vi "Receive Reference (FPGA).vi"() -> ()   [LabVIEW 2019]
uses:
  SubVIs/Sync/Sync Control.ctl
  SubVIs/Sync/Sync Measurements.ctl
  <instrlib>/_niInstr/DSP/v1/Shared/Public/IQ Impairments.ctl
  <instrlib>/_niInstr/DSP/v1/Shared/Public/Filter Coefficients.ctl
  Host/SubVIs/Low-level/TypeDefs/Gain Setting.ctl
  <instrlib>/niMmWave/ni3620/Config/v1/FPGA/Public/Typedefs/TX1 RX1 Port.ctl
  <vilib>/Platform/TimedLoop/XDataNode/timing_clust.ctl
  <vilib>/Platform/TimedLoop/XDataNode/nitl_modes.ctl
  <vilib>/Platform/TimedLoop/XDataNode/wakeup.ctl
  <vilib>/rvi/Emulation/niFpgaSctlEmulationGetInTimedLoop.vi
  <vilib>/rvi/Emulation/niFpgaEmulationReportErrorSimple.vi
  <vilib>/rvi/Emulation/niFpgaGetClockAttributes.vi
  <vilib>/rvi/Emulation/niFpgaCriticalErrorInLSC.vi
  <vilib>/rvi/Emulation/niFpgaProcessEmulError.vi
  <vilib>/rvi/eio/common/nirviEmuTemplateMethod_errors.vi
  SubVIs/Misc/Globals.vi
  <instrlib>/_niInstr/Data Formatting/v1/FPGA/Private/Convert/U8 array to Boolean Array.vi
  <vilib>/rvi/Emulation/niFpgaEmulationIsFPGAContextNoSignature.vi
  <vilib>/rvi/errors/niFpgaSetErrorForExecOnDevCompSimple.vi
  <vilib>/rvi/eio/common/nirviEmuReportErrorAndStop.vi
  <vilib>/rvi/DataTransferAndStorage/Container/Common/niFpgaContainerGetUniqueNameForEmu.vi
  <vilib>/rvi/FIFO/Fifo_Resource/nirvififoEmulationSetSize.vi
  <vilib>/rvi/FIFO/Fifo_Resource/nirviFifoEmulationQueueMgr.vi
  <instcachedir>/0/nirviFifoEmulationQueueMgr_E5CAEC123FF24DC58D834DCA3CDAA9B5.lvgen/nirviFifoEmulationQueueMgr_E5CAEC123FF24DC58D834DCA3CDAA9B5_008.vi
  <vilib>/rvi/FIFO/Fifo_Resource/nirvififoEmulationDetermineInputValidOut.vi
  <vilib>/rvi/FIFO/Fifo_Resource/nirvififoEmulationCreateLock.vi
  <vilib>/rvi/FIFO/Fifo_Resource/nirvififoEmulationObtainLock.vi
  <vilib>/rvi/FIFO/Fifo_Resource/nirvififoEmulationReleaseLock.vi
  <vilib>/rvi/occurrence/nirviWaitOnOccurrenceBase.vi
  <vilib>/rvi/errors/nirviReportUnexpectedCaseInternalError.vi
  <vilib>/rvi/errors/nirviReportUnexpectedCaseInternalError (U32).vi
  <vilib>/rvi/interface/RandomDataEmulation/nirviRandomDataMultiElementFPGAFIFO.vi
  <instcachedir>/0/nirviRandomDataMultiElementFPGAFIFO_1ED88BA00AC641F388A9B1FAA20E354D.lvgen/nirviRandomDataMultiElementFPGAFIFO_1ED88BA00AC641F388A9B1FAA20E354D_003.vi
  <vilib>/rvi/interface/RandomDataEmulation/niFpgaRandomDataHandleErrors.vi
  <instrlib>/_niInstr/Basic Elements/v1/FPGA/Private/Count Down U32.vi
  <instrlib>/_niInstr/Basic Elements/v1/FPGA/Private/Count Up U8.vi
  <vilib>/rvi/DataTransferAndStorage/Container/Common/niFpgaContainerSetEmuInfo.vi
  <vilib>/Utility/error.llb/Clear Errors.vi
  <vilib>/Platform/TimedLoop/XDataNode/XDataNode.xnode
  <vilib>/eio/EIONode/EIONode.xnode
  <vilib>/eio/EIOMethodNode/EIOMethodNode.xnode
  <vilib>/rvi/DataTransferAndStorage/Container/XNode/niFpgaContainer.xnode
  <vilib>/rvi/FIFO/Fifo_Resource/nirvififoEmulationWrite.vi
  <vilib>/rvi/interface/RandomDataEmulation/nirviRandomDataFpgaMultiElementTemplate.vi
  <vilib>/rvi/LocalResourceManager/LocalResourceManager.xnode
  <vilib>/rvi/FIFO/Fifo_Resource/nirvififoEmulationRead.vi
  <vilib>/Platform/TimedLoop/XDataNode/XDNodeRunTimeDep.lvlib
  <instrlib>/_niInstr/Basic Elements/v1/FPGA/niInstr Basic Elements v1 FPGA.lvlib
  <instrlib>/_niInstr/Data Formatting/v1/FPGA/niInstr Data Formatting v1 FPGA.lvlib
  <instrlib>/niMmWave/ni3620/Config/v1/FPGA/niMmWave Config v1 FPGA.lvlib
  <instrlib>/_niInstr/DSP/v1/Shared/niInstr DSP v1 Shared.lvlib
panel:
  in  "sync.master reset listen":bool
  in  "sync.counter reset enable":bool
  in  "20 kHz tclk parameters":T1
  out "tclk value":u16
  in  "gain ranging.enable port config":bool
  out "port 5.debug info":T2
  out "port 5.rx fifo overflow":bool
  in  "port 5.rx fifo overflow clear":bool
  in  "aurora.read port 5":bool
  out "port 4.rx fifo overflow":bool
  in  "port 4.rx fifo overflow clear":bool
  out "port 4.debug info":T2
  in  "aurora.read port 4":bool
  in  "gain ranging.enable coarse gain ranging":bool
  in  "gain ranging.enable fine gain ranging":bool
  in  "gain ranging.coarse gain values":fxp<+/-,16,12>[](array[numeric])=[0.0, 0.0, 0.0, 0.0]
  in  "table info":T3
  in  "gain ranging.manual setting":T6
  in  "gain ranging.setting list step":T7
  in  "gain ranging.enable":bool
  in  "gain ranging.dwell time (cycles)":u32=4800
  in  "rxjesd.control":T8
  out "rxjesd.status":T9
  in  "filter.enable":bool
  in  "filter.coefficients":T10
  in  "cal.correction":T12={"sample delay"={"I delay"=0.0, "Q delay"=0.0}, "fractional delay"={"enable"=FALSE, "coef write"=FALSE, "coef data"=0.0}, "impairments"={"inline gain I"=0.9999923706054688, "inline gain Q"=0.9999923706054688, "cross gain I"=0.0, "cross gain Q"=0.0, "pre-gain offset I"=0.0, "pre-gain offset Q"=0.0, "post-gain offset I"=0.0, "post-gain offset Q"=0.0}, "iq inversion"={"invert I"=FALSE, "invert Q"=FALSE}}
  out "sync.measurements":T13
  in  "sync.parameters":T15
  in  "acq.length":u32=1024
  out "aurora.fifo 1 overflow":bool
  in  "aurora.reset trigger":bool=TRUE
  out "aurora.fifo 0 overflow":bool
  in  "aurora.write":bool
  in  "aurora.fifo overflow clear":bool
  out "clocks valid":bool[](array[boolean])
  in  "cal.acquisition":T16={"acq length"=1024, "trigger type"=enum."software", "software trigger"=FALSE, "reset trigger detect"=FALSE}
  in  "sync.use synced trigger":bool
  in  "sync.trigger":bool
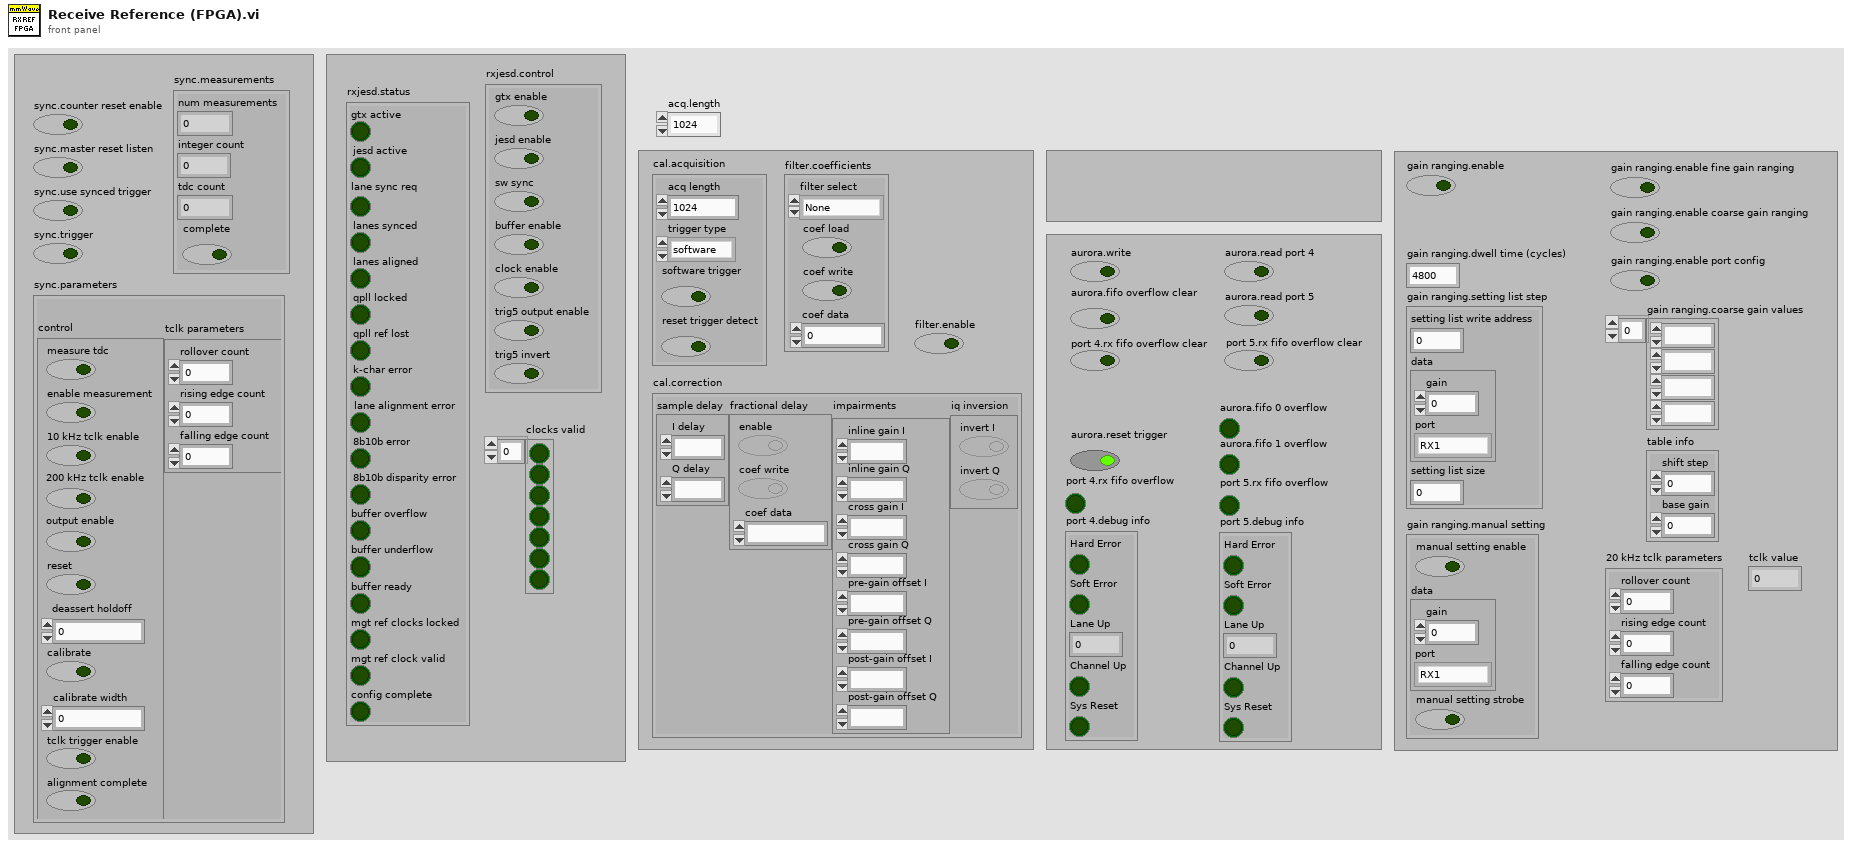
[diagram p1: front panel]
types:
  T1 = cluster{"rollover count":u16, "rising edge count":u16, "falling edge count":u16}
  T2 = cluster{"Hard Error":bool, "Soft Error":bool, "Lane Up":fxp<+,4,4>, "Channel Up":bool, "Sys Reset":bool}
  T3 = cluster{"shift step":i16, "base gain":fxp<+/-,16,12>}
  T4 = typedef "gain setting.ctl" = cluster{"gain":fxp<+/-,16,12>, "port":T5}
  T5 = typedef "TX1 RX1 Port.ctl" = enum8{"RX1", "TX1/RX2"}
  T6 = cluster{"manual setting enable":bool, "data":T4, "manual setting strobe":bool}
  T7 = cluster{"setting list write address":u32, "data":T4, "setting list size":u16}
  T8 = cluster{"gtx enable":bool, "jesd enable":bool, "sw sync":bool, "buffer enable":bool, "clock enable":bool, "trig5 output enable":bool, "trig5 invert":bool}
  T9 = cluster{"gtx active":bool, "jesd active":bool, "lane sync req":bool, "lanes synced":bool, "lanes aligned":bool, "qpll locked":bool, "qpll ref lost":bool, "k-char error":bool, "lane alignment error":bool, "8b10b error":bool, "8b10b disparity error":bool, "buffer overflow":bool, "buffer underflow":bool, "buffer ready":bool, "mgt ref clocks locked":bool, "mgt ref clock valid":bool, "config complete":bool}
  T10 = typedef "niInstr DSP v1 Shared.lvlib/Filter Coefficients.ctl" = cluster{"filter select":enum8{"None", "I Inline", "I Cross", "Q Cross", "Q Inline"}, "coef load":bool, "coef write":bool, "coef data":fxp<+/-,18,1>}
  T11 = typedef "niInstr DSP v1 Shared.lvlib/IQ Impairments.ctl" = cluster{"inline gain I":fxp<+/-,18,1>, "inline gain Q":fxp<+/-,18,1>, "cross gain I":fxp<+/-,18,1>, "cross gain Q":fxp<+/-,18,1>, "pre-gain offset I":fxp<+/-,18,1>, "pre-gain offset Q":fxp<+/-,18,1>, "post-gain offset I":fxp<+/-,18,1>, "post-gain offset Q":fxp<+/-,18,1>}
  T12 = cluster{"sample delay":cluster{"I delay":fxp<+,13,13>, "Q delay":fxp<+,13,13>}, "fractional delay":cluster{"enable":bool, "coef write":bool, "coef data":fxp<+/-,18,1>}, "impairments":T11, "iq inversion":cluster{"invert I":bool, "invert Q":bool}}
  T13 = typedef "Sync Measurements.ctl" = cluster{"num measurements":u16, "integer count":u16, "tdc count":u16, "complete":bool}
  T14 = typedef "Sync Control.ctl" = cluster{"measure tdc":bool, "enable measurement":bool, "10 kHz tclk enable":bool, "200 kHz tclk enable":bool, "output enable":bool, "reset":bool, "deassert holdoff":u8, "calibrate":bool, "calibrate width":u8, "tclk trigger enable":bool, "alignment complete":bool}
  T15 = cluster{"control":T14, "tclk parameters":cluster{"rollover count":u16, "rising edge count":u16, "falling edge count":u16}}
  T16 = cluster{"acq length":u16, "trigger type":enum16{"software", "external", "rising zero", "falling zero"}, "software trigger":bool, "reset trigger detect":bool}
  T17 = cluster{"m_axis_tvalid":refnum<k21>, "m_axis_tdata_0":refnum<k21>, "m_axis_tdata_1":refnum<k21>, "m_axis_tdata_2":refnum<k21>, "m_axis_tdata_3":refnum<k21>}
  T18 = cluster{"s_axis_tvalid":refnum<k21>, "s_axis_tdata_0":refnum<k21>, "s_axis_tdata_1":refnum<k21>, "s_axis_tdata_2":refnum<k21>, "s_axis_tdata_3":refnum<k21>, "s_axis_tready":refnum<k21>}
  T19 = typedef "Sync Resources.ctl" = cluster{"tdc assert":refnum<k21>, "tdc deassert":refnum<k21>, "tdc count":refnum<k21>, "control":refnum<k21>, "integer count":refnum<k21>}
  T20 = typedef "XDNodeRunTimeDep.lvlib/timing_clust.ctl" = cluster{"Expected End [f-1]":u64, "Actual End [f-1]":u64, "Finished Late? [f-1]":bool, "Expected End [i-1]":u64, "Actual End [i-1]":u64, "Finished Late? [i-1]":bool, "Expected Start [i]":u64, "Actual Start [i]":u64, "Expected Start [f]":u64, "Actual Start [f]":u64, "Source Name":string, "Structure Name":string, "Period":i64, "Deadline":i64, "Offset":i64, "Start":i64, "Priority":i32, "Timeout":i32, "Mode":T21, "Wakeup Reason":T22, "Error":errorcluster, "Source Type":string, "Secondary Source Type":string, "Global End Time":u64, "Global Start Time":u64, "Frame Duration":u64, "Iteration Duration":u64, "Assigned CPU":i32, "I/O Scan Engine Mode":u32}
  T21 = typedef "XDNodeRunTimeDep.lvlib/nitl_modes.ctl" = enum32{"No Change", "Process missed periods, maintain original phase", "Discard missed periods, maintain original phase", "Process missed periods, ignore original phase", "Discard missed periods, ignore original phase"}
  T22 = typedef "XDNodeRunTimeDep.lvlib/wakeup.ctl" = enum32{"Normal", "Aborted", "Asynchronous wakeup", "Timing source error", "Timed loop error", "Timeout"}
  T23 = cluster{"disable TClk measure":bool, "output enable":bool, "output value":bool}
  T24 = typedef "niInstr DSP v1 Shared.lvlib/IQ Data.ctl" = cluster{"I":fxp<+/-,18,1>, "Q":fxp<+/-,18,1>, "overflow":bool}
  T25 = typedef "AXI4-Stream Reader FXP64x4 Resources.ctl" = cluster{"AXI4-Stream Reader Resources":cluster{"Use TREADY":bool, "Use TLAST":bool, "TLAST":refnum<k21>, "TREADY":refnum<k21>, "TVALID":refnum<k21>, "Use TKEEP":bool, "Use TSTRB":bool, "Use TUSER":bool}, "TDATA Resources":cluster{"TDATA_0":refnum<k21>, "TDATA_1":refnum<k21>, "TDATA_2":refnum<k21>, "TDATA_3":refnum<k21>}, "TKEEP":refnum<k21>, "TSTRB":refnum<k21>}
  T26 = typedef "AXI4-Stream Writer FXP64x4 Resources.ctl" = cluster{"Writer Resources":cluster{"Use TREADY":bool, "Use TLAST":bool, "TLAST":refnum<k21>, "TREADY":refnum<k21>, "TVALID":refnum<k21>, "Use TSTRB":bool, "Use TKEEP":bool, "Use TUSER":bool}, "TDATA Resources":cluster{"TDATA_0":refnum<k21>, "TDATA_1":refnum<k21>, "TDATA_2":refnum<k21>, "TDATA_3":refnum<k21>}, "TKEEP":refnum<k21>, "TSTRB":refnum<k21>}
  T27 = cluster{"Hard Error":refnum<k21>, "Soft Error":refnum<k21>, "Lane Up":refnum<k21>, "Channel Up":refnum<k21>, "Sys Reset":refnum<k21>}
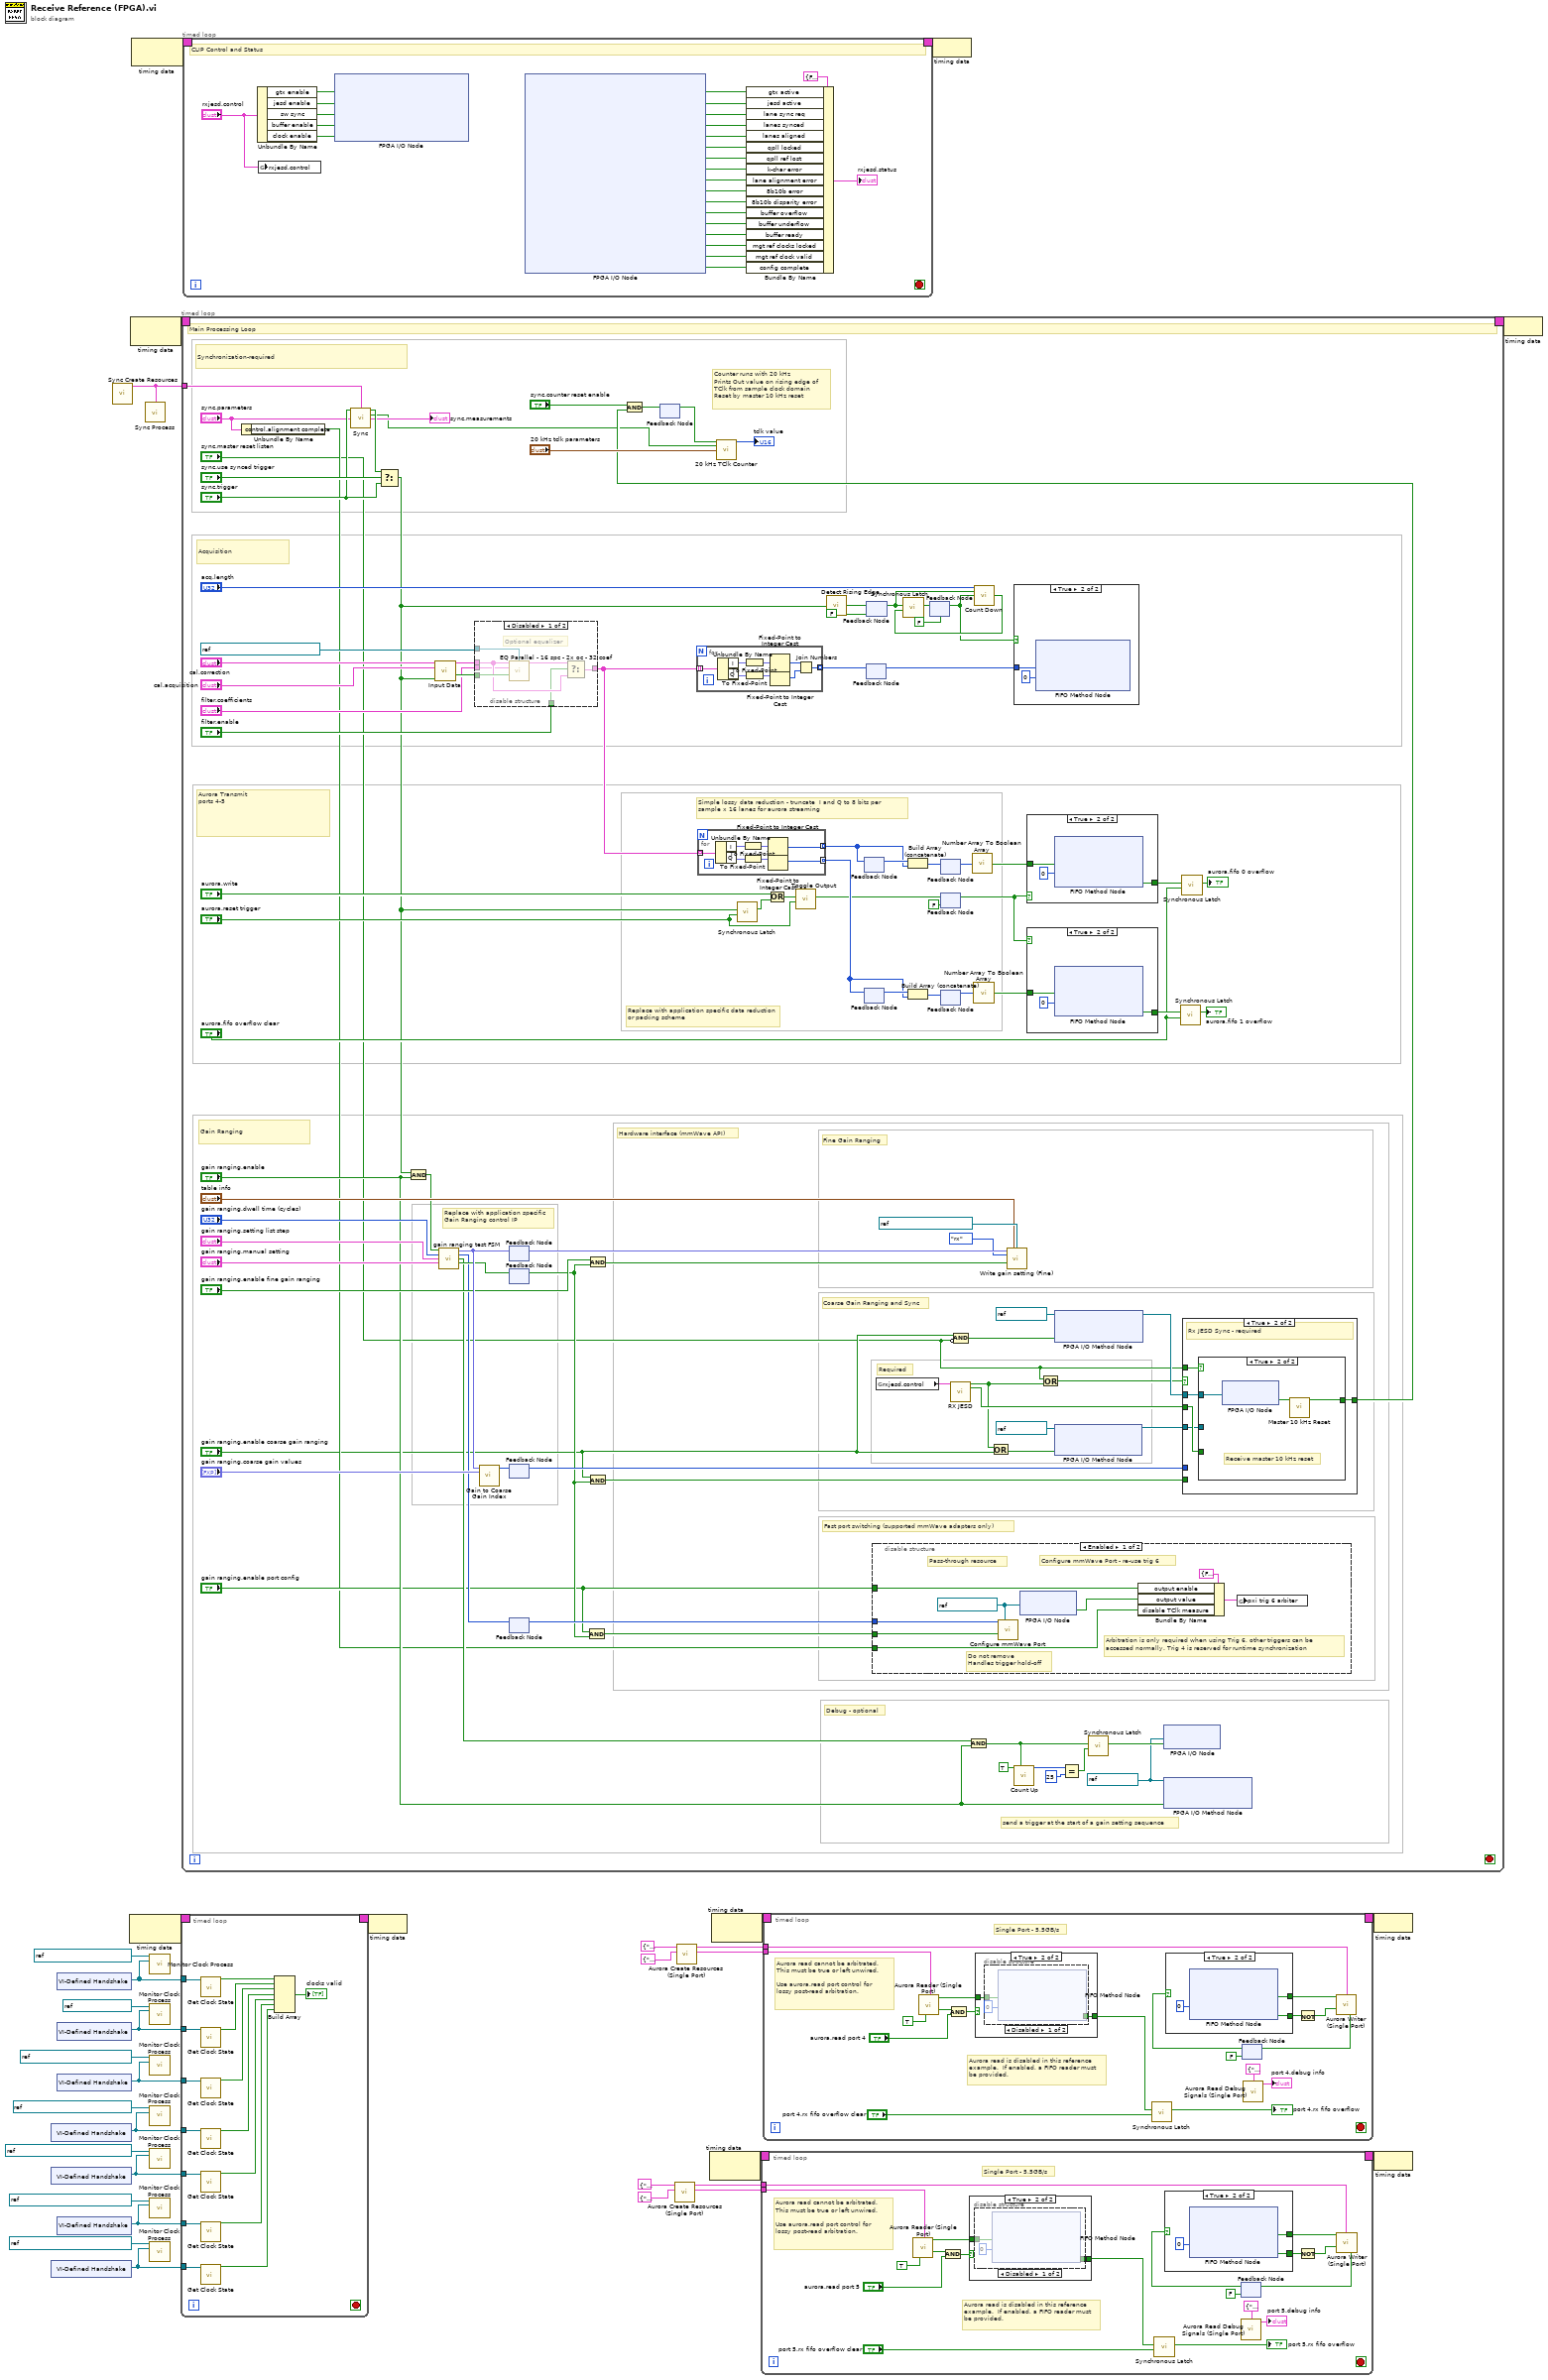
[diagram p0: block diagram]
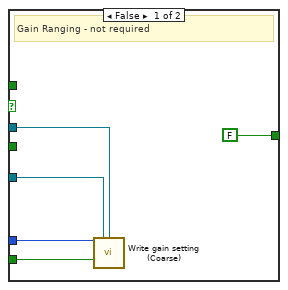
[diagram p2: hidden frame]
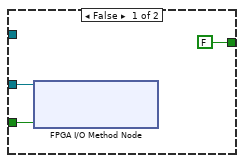
[diagram p3: hidden frame]
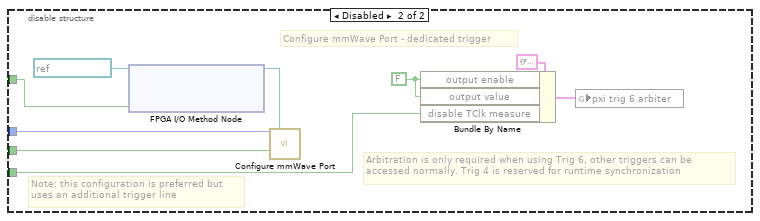
[diagram p4: hidden frame]
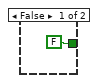
[diagram p7: hidden frame]
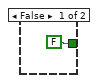
[diagram p8: hidden frame]
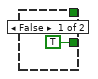
[diagram p9: hidden frame]
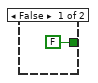
[diagram p10: hidden frame]
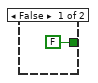
[diagram p12: hidden frame]
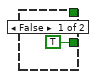
[diagram p14: hidden frame]
diagram:
  n1 = xnode "VI-Defined Handshake"() -> ("Handshake Out"=w10:refnum<k21>)
  n2 = xnode "VI-Defined Handshake"() -> ("Handshake Out"=w11:refnum<k21>)
  n3 = xnode "VI-Defined Handshake"() -> ("Handshake Out"=w18:refnum<k21>)
  n4 = xnode "VI-Defined Handshake"() -> ("Handshake Out"=w25:refnum<k21>)
  n5 = xnode "VI-Defined Handshake"() -> ("Handshake Out"=w24:refnum<k21>)
  n6 = xnode "VI-Defined Handshake"() -> ("Handshake Out"=w20:refnum<k21>)
  n7 = xnode "VI-Defined Handshake"() -> ("Handshake Out"=w21:refnum<k21>)
  n8 = call "Sync Create Resources.vi"() -> ("sync.resources"=w29:T19)  [unwired: 15 in]
  n9 = node-c288() -> (w28:T20)  [unwired: 1 in]
  n10 = node-c288() -> (w31:T20)  [unwired: 1 in]
  n11 = node-c288() -> (w33:T20)  [unwired: 1 in]
  n12 = call "Sync Process.vi"("sync.resources"=w29) -> ()  [unwired: 15 in]
  n13 = call "Monitor Clock Process.vi"("clock name"=refnum<k21> "40 MHz Onboard Clock", "handshake"=w25) -> ()  [unwired: 14 in]
  n14 = call "Monitor Clock Process.vi"("clock name"=refnum<k21> "100 MHz Clock", "handshake"=w24) -> ()  [unwired: 14 in]
  n15 = call "Monitor Clock Process.vi"("clock name"=refnum<k21> "7902R IO Socket\\SampleClk", "handshake"=w20) -> ()  [unwired: 14 in]
  n16 = call "Monitor Clock Process.vi"("clock name"=refnum<k21> "7902R IO Socket\\SampleClkx2", "handshake"=w10) -> ()  [unwired: 14 in]
  n17 = call "Monitor Clock Process.vi"("clock name"=refnum<k21> "7902R IO Socket\\SampleClkDiv2", "handshake"=w11) -> ()  [unwired: 14 in]
  n18 = call "Monitor Clock Process.vi"("clock name"=refnum<k21> "7902R IO Socket\\Port4_UserClk", "handshake"=w21) -> ()  [unwired: 14 in]
  n19 = call "Monitor Clock Process.vi"("clock name"=refnum<k21> "7902R IO Socket\\Port5_UserClk", "handshake"=w18) -> ()  [unwired: 14 in]
  n20 = timed-loop {
    timing: w28 -> [_]
    timing-out: [_] -> w27
    tunnel: w25 -> [w48]
    tunnel: w24 -> [w47]
    tunnel: w20 -> [w42]
    tunnel: w21 -> [w43]
    tunnel: w18 -> [w40]
    tunnel: w10 -> [w38]
    tunnel: w11 -> [w39]
    stop <- _ stop-if-true
    n21 = call "Get Clock State.vi"("handshake in"=w48) -> ("clock valid"=w46:bool)  [unwired: 14 in]
    n22 = call "Get Clock State.vi"("handshake in"=w47) -> ("clock valid"=w45:bool)  [unwired: 14 in]
    n23 = call "Get Clock State.vi"("handshake in"=w42) -> ("clock valid"=w41:bool)  [unwired: 14 in]
    n24 = call "Get Clock State.vi"("handshake in"=w38) -> ("clock valid"=w35:bool)  [unwired: 14 in]
    n25 = call "Get Clock State.vi"("handshake in"=w39) -> ("clock valid"=w34:bool)  [unwired: 14 in]
    n26 = call "Get Clock State.vi"("handshake in"=w43) -> ("clock valid"=w36:bool)  [unwired: 14 in]
    n27 = call "Get Clock State.vi"("handshake in"=w40) -> ("clock valid"=w37:bool)  [unwired: 14 in]
    n28 = Build Array(w46, w45, w41, w35, w34, w36, w37) -> (→"clocks valid":bool[])
  }
  n29 = timed-loop {
    timing: w31 -> [_]
    timing-out: [_] -> w30
    tunnel: w29 -> [w123]
    stop <- _ stop-if-true
    w80 = refnum<k21> "PXI_Trig3" ("FPGA I/O In")
    # "Counter runs with 20 kHz\nPrints Out value on rising edge of \nTClk from sample clock domain\nReset by master 10 kHz reset"
    # "Replace with application specific Gain Ranging control IP"
    # "Simple lossy data reduction - truncate  I and Q to 8 bits per sample x 16 lanes for aurora streaming"
    # "Replace with application specific data reduction or packing scheme"
    # "Debug - optional"
    # "Fast port switching (supported mmWave adapters only)"
    # "Coarse Gain Ranging and Sync"
    # "Fine Gain Ranging"
    # "Hardware interface (mmWave API)"
    # "Gain Ranging"
    # "Aurora Transmit\nports 4-5"
    # "Acquisition"
    # "Synchronization-required"
    # "Required"
    # "send a trigger at the start of a gain setting sequence"
    # "Main Processing Loop"
    n30 = Unbundle By Name("sync.parameters") -> ("control.alignment complete"=w63:bool)
    n31 = call "Sync.vi"("trigger"="sync.trigger", "sync.resources"=w123, "sync.parameters"="sync.parameters") -> ("synced trigger"=w124:bool, "tclk"=w54:bool, "sync measurements"=→"sync.measurements":T13)  [unwired: 10 in]
    n32 = Select(t=w124, s="sync.use synced trigger", f="sync.trigger") -> (s? t:f=w101:bool)
    n33 = And(x=w101, y="gain ranging.enable") -> (x .and. y?=w78:bool)
    n34 = call "Input Data.vi"("cal parameters"="cal.correction", "acq parameters"="cal.acquisition", "external trigger"=w101) -> ("adc data"=w108:T24[], "output valid"=w110:bool)  [unwired: 11 in]
    n35 = call "gain ranging test FSM.vi"("gain ranging.start sequence"=w78, "gain ranging.dwell time (cycles)"="gain ranging.dwell time (cycles)", "gain ranging.gain setting list"="gain ranging.setting list step", "gain ranging.manual request"="gain ranging.manual setting") -> ("gain ranging.gain setting"=w95:fxp<+/-,16,12>, "gain ranging.TX1/RX1 Port Value"=w88:T5, "gain ranging.start of sequence"=w86:bool, "gain ranging.gain setting valid"=w90:bool)  [unwired: 8 in]
    n36 = disable-structure shown="Disabled" {
      disable-tunnel: w110 -> [w187 _]
      disable-tunnel: [w185 w188] -> w109
      disable-tunnel: w108 -> [w184 w188]
      disable-tunnel: "filter.coefficients" -> [w183 _]
      disable-tunnel: "filter.enable" -> [w182 _]
      disable-tunnel: refnum<k21> "7902R IO Socket\\SampleClkx2" ("clock x2") -> [w181 _]
      frame Disabled {
        # "Optional equalizer"
        n37 = call "EQ Parallel - 16 spc - 2x oc - 32 coef.vi"("data in"=w184, "clock x2"=w181, "filter coefficients"=w183, "input valid"=w187) -> ("data out"=w186:T24[])  [unwired: 9 in, 2 out]
        n38 = Select(t=w186, s=w182, f=w184) -> (s? t:f=w185:T24[])
      }
      frame Enabled {
      }
    }
    n39 = call "Gain to Coarse Gain Index.vi"("gain setting"=w95, "coarse gain values"="gain ranging.coarse gain values") -> ("coarse gain index"=w93:u32)  [unwired: 13 in]
    n40 = feedback #1() -> (w94:fxp<+/-,16,12>)  [unwired: 1 in]
    n41 = feedback-in #1(w95) -> ()
    n42 = feedback #2() -> (w68:bool)  [unwired: 1 in]
    n43 = feedback-in #2(w90) -> ()
    n44 = feedback #3() -> (w71:u32)  [unwired: 1 in]
    n45 = feedback-in #3(w93) -> ()
    n46 = feedback #4() -> (w76:T5)  [unwired: 1 in]
    n47 = feedback-in #4(w88) -> ()
    n48 = And(x="gain ranging.enable port config", y=w68) -> (x .and. y?=w67:bool)
    n49 = And(x="gain ranging.enable fine gain ranging", y=w68) -> (x .and. y?=w89:bool)
    n50 = And(x="gain ranging.enable coarse gain ranging", y=w68) -> (x .and. y?=w70:bool)
    n51 = feedback #5() -> (w55:bool)  [unwired: 1 in]
    n52 = for {
      tunnel: [w196] -> w112 mode=indexing
      tunnel: w109 -> [w195] mode=indexing
      n53 = Unbundle By Name(w195) -> ("I"=w194:fxp<+/-,18,1>, "Q"=w193:fxp<+/-,18,1>)
      n54 = To Fixed-Point(number=w194) -> (fixed-point=w198:fxp<+/-,16,1>)  [unwired: 1 in]
      n55 = To Fixed-Point(number=w193) -> (fixed-point=w197:fxp<+/-,16,1>)  [unwired: 1 in]
      n56 = Fixed-Point to Integer Cast(1:w198) -> (0:w192:i16)
      n57 = Fixed-Point to Integer Cast(1:w197) -> (0:w191:i16)
      n58 = Join Numbers(hi=w192, lo=w191) -> ((hi.lo)=w196:u32)
    }
    n59 = for {
      tunnel: w109 -> [w211] mode=indexing
      tunnel: [w208] -> w117 mode=indexing
      tunnel: [w207] -> w120 mode=indexing
      n60 = Unbundle By Name(w211) -> ("I"=w210:fxp<+/-,18,1>, "Q"=w209:fxp<+/-,18,1>)
      n61 = To Fixed-Point(number=w210) -> (fixed-point=w213:fxp<+/-,8,1>)  [unwired: 1 in]
      n62 = To Fixed-Point(number=w209) -> (fixed-point=w212:fxp<+/-,8,1>)  [unwired: 1 in]
      n63 = Fixed-Point to Integer Cast(1:w213) -> (0:w208:i8)
      n64 = Fixed-Point to Integer Cast(1:w212) -> (0:w207:i8)
    }
    n65 = call "20 kHz TClk Counter.vi"("master 10 kHz reset"=w55, "tclk"=w54, "20 kHz tclk parameters"="20 kHz tclk parameters") -> ("tclk offset value"=→"tclk value":u16)  [unwired: 12 in]
    n66 = call <instrlib>:"Synchronous Latch.vi"("clear"="aurora.reset trigger", "set"=w101) -> ("out"=w140:bool)  [unwired: 9 in]
    n67 = Or(x="aurora.write", y=w140) -> (x .or. y?=w115:bool)
    n68 = call <instrlib>:"Toggle Output.vi"("clear"="aurora.reset trigger", "toggle"=w115) -> ("output"=w114:bool)  [unwired: 9 in]
    n69 = call <instrlib>:"Detect Rising Edge.vi"("signal"=w101) -> ("edge detected"=w129:bool)  [unwired: 14 in]
    n70 = feedback #6() -> (w118:i8[])  [unwired: 1 in]
    n71 = feedback-in #6(w117) -> ()
    n72 = feedback #7() -> (w121:i8[])  [unwired: 1 in]
    n73 = feedback-in #7(w120) -> ()
    n74 = feedback #8() -> (w128:u32[])  [unwired: 1 in]
    n75 = feedback-in #8(w112) -> ()
    n76 = feedback #9(FALSE ("edge detected")) -> (w130:bool)
    n77 = feedback-in #9(w129) -> ()
    n78 = disable-structure shown="Enabled" {
      disable-tunnel: w67 -> [w169 w178]
      disable-tunnel: w76 -> [w168 w177]
      disable-tunnel: "gain ranging.enable port config" -> [w166 w174]
      disable-tunnel: w63 -> [w164 w172]
      frame Enabled {
        w165 = refnum<k21> "PXIe_DStarC" ("FPGA I/O In")
        # "Do not remove\nHandles trigger hold-off"
        # "Configure mmWave Port - re-use trig 6"
        # "Pass-through resource"
        # "Arbitration is only required when using Trig 6, other triggers can be accessed normally. Trig 4 is reserved for runtime synchronization"
        n79 = call <instrlib>:"Configure mmWave Port.vi"("port"=w168, "pxi trigger"=w165, "input valid"=w169) -> ()  [unwired: 12 in, 1 out]
        n80 = xnode "FPGA I/O Node"("FPGA I/O In"=w165) -> ("I/O Item"=w167:bool)  [unwired: 1 out]
        n81 = Bundle By Name(cluster=T23 {"disable TClk measure"=FALSE, "output enable"=FALSE, "output value"=FALSE} ("pxi trig 6 arbiter"), "output enable"=w166, "output value"=w167, "disable TClk measure"=w164) -> (w170:T23)
        n82 = global write "Globals.vi" "pxi trig 6 arbiter"(w170) -> ()
      }
      frame Disabled {
        w176 = FALSE ("disable TClk measure")
        # "Note: this configuration is preferred but \nuses an additional trigger line"
        # "Configure mmWave Port - dedicated trigger"
        # "Arbitration is only required when using Trig 6, other triggers can be accessed normally. Trig 4 is reserved for runtime synchronization"
        n83 = xnode "FPGA I/O Method Node"("FPGA I/O In"=refnum<k21> "PXI_Trig0" ("pxi trigger 1"), "Enable"=w174) -> ("FPGA I/O Out"=w175:refnum<k21>)
        n84 = call <instrlib>:"Configure mmWave Port.vi"("port"=w177, "pxi trigger"=w175, "input valid"=w178) -> ()  [unwired: 12 in, 1 out]
        n85 = Bundle By Name(cluster=T23 {"disable TClk measure"=FALSE, "output enable"=FALSE, "output value"=FALSE} ("pxi trig 6 arbiter"), "output enable"=w176, "output value"=w176, "disable TClk measure"=w172) -> (w179:T23)
        n86 = global write "Globals.vi" "pxi trig 6 arbiter"(w179) -> ()
      }
    }
    n87 = global read "Globals.vi" "rxjesd.control"() -> (w97:T8)
    n88 = Build Array (concatenate)(w118, w117) -> (w116:i8[])
    n89 = Build Array (concatenate)(w121, w120) -> (w119:i8[])
    n90 = feedback #10(FALSE ("out")) -> (w125:bool)
    n91 = feedback #11() -> (w142:i8[])  [unwired: 1 in]
    n92 = feedback-in #11(w116) -> ()
    n93 = feedback #12(FALSE) -> (w138:bool)
    n94 = feedback-in #12(w114) -> ()
    n95 = feedback #13() -> (w137:i8[])  [unwired: 1 in]
    n96 = feedback-in #13(w119) -> ()
    n97 = call "RX JESD.vi"("rxjesd.control"=w97) -> ("trigger output enable"=w53:bool, "trigger value"=w73:bool)  [unwired: 13 in]
    n98 = Compound Arithmetic op=AND("gain ranging.enable coarse gain ranging", invert "sync.master reset listen") -> (w61:bool)
    n99 = And(x=w86, y="gain ranging.enable") -> (x .and. y?=w79:bool)
    n100 = call-poly <instrlib>:"Number Array To Boolean Array.vi"("data in"=w142) -> ("data out"=w145:bool[])  [unwired: 14 in]
    n101 = call-poly <instrlib>:"Number Array To Boolean Array.vi"("data in"=w137) -> ("data out"=w136:bool[])  [unwired: 14 in]
    n102 = call-poly <instrlib>:"Count Down.vi"("count in"="acq.length", "load"=w130, "decrement"=w125) -> ("terminal count"=w126:bool)  [unwired: 11 in, 1 out]
    n103 = call <instrlib>:"Synchronous Latch.vi"("clear"=w126, "set"=w130) -> ("out"=w127:bool)  [unwired: 9 in]
    n104 = feedback-in #10(w127) -> ()
    n105 = Or(x=w53, y="gain ranging.enable coarse gain ranging") -> (x .or. y?=w69:bool)
    n106 = call <instrlib>:"Write gain setting (Fine).vi"("gain"=w94, "table info"="table info", "P2P Writer FIFO"=refnum<k21> "P2P FIFO to PXIe-3620" ("FIFO In"), "direction"=enum8{"rx", "tx"}."rx", "input valid"=w89) -> ()  [unwired: 10 in, 1 out]
    n107 = case shown="True" w125 {
      tunnel: w128 -> [_ w190]
      frame False {
      }
      frame True {
        n108 = xnode ("FIFO Method Node")("Element"=w190, "Timeout"=0) -> ()  [unwired: 1 in, 2 out]
      }
    }
    n109 = call-poly <instrlib>:"Count Up.vi"("increment"=TRUE, "reset"=w79) -> ("count out"=w84:u8)  [unwired: 13 in]
    n110 = case shown="True" w138 {
      tunnel: [FALSE ("Timed Out?") w206] -> w143
      tunnel: w145 -> [_ w205]
      frame False {
      }
      frame True {
        n111 = xnode ("FIFO Method Node")("Element"=w205, "Timeout"=0) -> ("Timed Out?"=w206:bool)  [unwired: 1 in, 1 out]
      }
    }
    n112 = case shown="True" w138 {
      tunnel: [FALSE ("Timed Out?") w202] -> w134
      tunnel: w136 -> [_ w201]
      frame False {
      }
      frame True {
        n113 = xnode ("FIFO Method Node")("Element"=w201, "Timeout"=0) -> ("Timed Out?"=w202:bool)  [unwired: 1 in, 1 out]
      }
    }
    n114 = Or(x="sync.master reset listen", y=w53) -> (x .or. y?=w52:bool)
    n115 = xnode "FPGA I/O Method Node"("FPGA I/O In"=refnum<k21> "PXI_Trig5" ("pxi trigger 1"), "Enable"=w69) -> ("FPGA I/O Out"=w72:refnum<k21>)
    n116 = xnode "FPGA I/O Method Node"("FPGA I/O In"=refnum<k21> "PXI_Trig7" ("pxi trigger 1"), "Enable"=w61) -> ("FPGA I/O Out"=w74:refnum<k21>)
    n117 = Equal?(x=w84, y=u8 25) -> (x = y?=w82:bool)
    n118 = call <instrlib>:"Synchronous Latch.vi"("clear"=w82, "set"=w79) -> ("out"=w81:bool)  [unwired: 9 in]
    n119 = xnode "FPGA I/O Node"("I/O Item"=w81, "FPGA I/O In"=w80) -> ()  [unwired: 1 out]
    n120 = xnode "FPGA I/O Method Node"("FPGA I/O In"=w80, "Enable"="gain ranging.enable") -> ()  [unwired: 1 out]
    n121 = call <instrlib>:"Synchronous Latch.vi"("clear"="aurora.fifo overflow clear", "set"=w134) -> ("out"=→"aurora.fifo 1 overflow":bool)  [unwired: 9 in]
    n122 = call <instrlib>:"Synchronous Latch.vi"("clear"="aurora.fifo overflow clear", "set"=w143) -> ("out"=→"aurora.fifo 0 overflow":bool)  [unwired: 9 in]
    n123 = case shown="True" w52 {
      tunnel: w74 -> [w152 w153]
      tunnel: w73 -> [_ w157]
      tunnel: w72 -> [w151 w156]
      tunnel: w71 -> [w150 _]
      tunnel: w70 -> [w149 _]
      tunnel: [FALSE ("Master10k_Reset") w155] -> w58
      tunnel: "sync.master reset listen" -> [_ w154]
      frame False {
        # "Gain Ranging - not required"
        n124 = call <instrlib>:"Write gain setting (Coarse).vi"("fast jump table index"=w150, "pxi trigger 1"=w151, "pxi trigger 2"=w152, "input valid"=w149) -> ()  [unwired: 11 in, 1 out]
      }
      frame True {
        # "Rx JESD Sync - required"
        n125 = case shown="True" w154 {
          tunnel: w157 -> [w160 _]
          tunnel: w156 -> [w159 _]
          tunnel: [FALSE ("Master10k_Reset") w161] -> w155
          tunnel: w153 -> [_ w162]
          frame False {
            n126 = xnode "FPGA I/O Method Node"("FPGA I/O In"=w159, "Data"=w160) -> ()  [unwired: 1 out]
          }
          frame True {
            # "Receive master 10 kHz reset"
            n127 = xnode "FPGA I/O Node"("FPGA I/O In"=w162) -> ("I/O Item"=w163:bool)  [unwired: 1 out]
            n128 = call "Master 10 kHz Reset.vi"("I/O Item"=w163) -> ("master 10 kHz reset"=w161:bool)  [unwired: 10 in]
          }
        }
      }
    }
    n129 = And(x="sync.counter reset enable", y=w58) -> (x .and. y?=w57:bool)
    n130 = feedback-in #5(w57) -> ()
  }
  n131 = timed-loop {
    timing: w33 -> [_]
    timing-out: [_] -> w32
    stop <- _ stop-if-true
    # "CLIP Control and Status"
    n132 = Unbundle By Name("rxjesd.control") -> ("gtx enable"=w218:bool, "jesd enable"=w222:bool, "sw sync"=w221:bool, "buffer enable"=w220:bool, "clock enable"=w217:bool)
    n133 = global write "Globals.vi" "rxjesd.control"("rxjesd.control") -> ()
    n134 = xnode "FPGA I/O Node"("7902R IO Socket\\aGtxEnable"=w218, "7902R IO Socket\\aJesdEnable"=w222, "7902R IO Socket\\aSyncFromSw"=w221, "7902R IO Socket\\aBufferEnable"=w220, "7902R IO Socket\\aClkEnable"=w217) -> ()  [unwired: 5 in, 5 out]
    n135 = xnode "FPGA I/O Node"() -> ("7902R IO Socket\\aGtxActive"=w216:bool, "7902R IO Socket\\aJesdActive"=w239:bool, "7902R IO Socket\\aLaneSyncReq"=w238:bool, "7902R IO Socket\\aLanesSynced"=w237:bool, "7902R IO Socket\\aLanesAligned"=w236:bool, "7902R IO Socket\\aQpllLocked"=w235:bool, "7902R IO Socket\\aQpllRefLost"=w234:bool, "7902R IO Socket\\aKCharError"=w233:bool, "7902R IO Socket\\aLaneAlignError"=w232:bool, "7902R IO Socket\\a8b10bNotInTable"=w231:bool, "7902R IO Socket\\a8b10bDispError"=w230:bool, "7902R IO Socket\\aBufferOverflow"=w229:bool, "7902R IO Socket\\aBufferUnderflow"=w228:bool, "7902R IO Socket\\aBufferReady"=w227:bool, "7902R IO Socket\\MgtRefClks_Locked"=w226:bool, "7902R IO Socket\\MgtRefClks_Valid"=w225:bool, "7902R IO Socket\\sFrontEndConfig_Complete"=w224:bool)  [unwired: 17 in, 17 out]
    n136 = Bundle By Name(cluster=T9 {"gtx active"=FALSE, "jesd active"=FALSE, "lane sync req"=FALSE, "lanes synced"=FALSE, "lanes aligned"=FALSE, "qpll locked"=FALSE, "qpll ref lost"=FALSE, "k-char error"=FALSE, "lane alignment error"=FALSE, "8b10b error"=FALSE, "8b10b disparity error"=FALSE, "buffer overflow"=FALSE, "buffer underflow"=FALSE, "buffer ready"=FALSE, "mgt ref clocks locked"=FALSE, "mgt ref clock valid"=FALSE, "config complete"=FALSE} ("rxjesd.status 2"), "gtx active"=w216, "jesd active"=w239, "lane sync req"=w238, "lanes synced"=w237, "lanes aligned"=w236, "qpll locked"=w235, "qpll ref lost"=w234, "k-char error"=w233, "lane alignment error"=w232, "8b10b error"=w231, "8b10b disparity error"=w230, "buffer overflow"=w229, "buffer underflow"=w228, "buffer ready"=w227, "mgt ref clocks locked"=w226, "mgt ref clock valid"=w225, "config complete"=w224) -> (→"rxjesd.status":T9)
  }
  n137 = node-c288(w27) -> ()
  n138 = call "Aurora Create Resources (Single Port).vi"("RX CLIP Resources"=T17 {"m_axis_tvalid"="7902R IO Socket\\uPort5_m_axi_rx_tvalid", "m_axis_tdata_0"="7902R IO Socket\\uPort5_m_axi_rx_tdata_0", "m_axis_tdata_1"="7902R IO Socket\\uPort5_m_axi_rx_tdata_1", "m_axis_tdata_2"="7902R IO Socket\\uPort5_m_axi_rx_tdata_2", "m_axis_tdata_3"="7902R IO Socket\\uPort5_m_axi_rx_tdata_3"}, "TX CLIP Resources"=T18 {"s_axis_tvalid"="7902R IO Socket\\uPort5_s_axi_tx_tvalid", "s_axis_tdata_0"="7902R IO Socket\\uPort5_s_axi_tx_tdata_0", "s_axis_tdata_1"="7902R IO Socket\\uPort5_s_axi_tx_tdata_1", "s_axis_tdata_2"="7902R IO Socket\\uPort5_s_axi_tx_tdata_2", "s_axis_tdata_3"="7902R IO Socket\\uPort5_s_axi_tx_tdata_3", "s_axis_tready"="7902R IO Socket\\uPort5_s_axi_tx_tready"}) -> ("AXI4-Stream Reader FXP64x4"=w3:T25, "AXI4-Stream Writer FXP64x4"=w4:T26)  [unwired: 8 in]
  n139 = call "Aurora Create Resources (Single Port).vi"("RX CLIP Resources"=T17 {"m_axis_tvalid"="7902R IO Socket\\uPort4_m_axi_rx_tvalid", "m_axis_tdata_0"="7902R IO Socket\\uPort4_m_axi_rx_tdata_0", "m_axis_tdata_1"="7902R IO Socket\\uPort4_m_axi_rx_tdata_1", "m_axis_tdata_2"="7902R IO Socket\\uPort4_m_axi_rx_tdata_2", "m_axis_tdata_3"="7902R IO Socket\\uPort4_m_axi_rx_tdata_3"}, "TX CLIP Resources"=T18 {"s_axis_tvalid"="7902R IO Socket\\uPort4_s_axi_tx_tvalid", "s_axis_tdata_0"="7902R IO Socket\\uPort4_s_axi_tx_tdata_0", "s_axis_tdata_1"="7902R IO Socket\\uPort4_s_axi_tx_tdata_1", "s_axis_tdata_2"="7902R IO Socket\\uPort4_s_axi_tx_tdata_2", "s_axis_tdata_3"="7902R IO Socket\\uPort4_s_axi_tx_tdata_3", "s_axis_tready"="7902R IO Socket\\uPort4_s_axi_tx_tready"}) -> ("AXI4-Stream Reader FXP64x4"=w1:T25, "AXI4-Stream Writer FXP64x4"=w2:T26)  [unwired: 8 in]
  n140 = node-c288 ("Input Node")() -> (w6:T20)  [unwired: 1 in]
  n141 = node-c288() -> (w8:T20)  [unwired: 1 in]
  n142 = timed-loop {
    timing: w6 -> [_]
    timing-out: [_] -> w5
    tunnel: w4 -> [w248]
    tunnel: w3 -> [w252]
    stop <- _ stop-if-true
    # "Aurora read cannot be arbitrated. This must be true or left unwired.\n\nUse aurora.read port control for lossy post-read arbitration."
    # "Aurora read is disabled in this reference\nexample.  If enabled, a FIFO reader must\nbe provided."
    # "Single Port - 5.5GB/s"
    n143 = call "Aurora Reader (Single Port) .vi"("AXI4-Stream Reader FXP64x4"=w252, "ready for output"=TRUE) -> ("data"=w253:bool[], "output valid"=w246:bool)  [unwired: 12 in]
    n144 = And(x=w246, y="aurora.read port 5") -> (x .and. y?=w244:bool)
    n145 = case shown="True" w244 {
      tunnel: w253 -> [_ w267]
      tunnel: [FALSE ("Timed Out?") w266] -> w247
      frame False {
      }
      frame True {
        n146 = disable-structure shown="Disabled" {
          disable-tunnel: w267 -> [w270 _]
          disable-tunnel: [w269 _] -> w266
          frame Disabled {
            n147 = xnode ("FIFO Method Node")("Element"=w270, "Timeout"=0) -> ("Timed Out?"=w269:bool)  [unwired: 1 in, 1 out]
          }
          frame Enabled {
          }
        }
      }
    }
    n148 = call <instrlib>:"Synchronous Latch.vi"("clear"="port 5.rx fifo overflow clear", "set"=w247) -> ("out"=→"port 5.rx fifo overflow":bool)  [unwired: 9 in]
    n149 = feedback #14(FALSE ("ready for input")) -> (w255:bool)
    n150 = case shown="True" w255 {
      tunnel: [_ w264] -> w251
      tunnel: [TRUE ("Timed Out?") w263] -> w256
      frame False {
      }
      frame True {
        n151 = xnode ("FIFO Method Node")("Timeout"=0) -> ("Element"=w264:bool[], "Timed Out?"=w263:bool)  [unwired: 1 in, 1 out]
      }
    }
    n152 = call "Aurora Read Debug Signals (Single Port).vi"("Debug CLIP Resources"=T27 {"Hard Error"="7902R IO Socket\\uPort5_HardError", "Soft Error"="7902R IO Socket\\uPort5_SoftError", "Lane Up"="7902R IO Socket\\uPort5_LaneUp", "Channel Up"="7902R IO Socket\\uPort5_ChannelUp", "Sys Reset"="7902R IO Socket\\uPort5_sys_reset_out"}) -> ("Debug Info"=→"port 5.debug info":T2)  [unwired: 14 in]
    n153 = Not(x=w256) -> (.not. x?=w250:bool)
    n154 = call "Aurora Writer (Single Port).vi"("input data"=w251, "AXI4-Stream Writer FXP64x4"=w248, "input valid"=w250) -> ("ready for input"=w249:bool)  [unwired: 12 in]
    n155 = feedback-in #14(w249) -> ()
  }
  n156 = timed-loop {
    timing: w8 -> [_]
    timing-out: [_] -> w7
    tunnel: w2 -> [w290]
    tunnel: w1 -> [w275]
    stop <- _ stop-if-true
    # "Aurora read cannot be arbitrated. This must be true or left unwired.\n\nUse aurora.read port control for lossy post-read arbitration."
    # "Aurora read is disabled in this reference\nexample.  If enabled, a FIFO reader must\nbe provided."
    # "Single Port - 5.5GB/s"
    n157 = call "Aurora Reader (Single Port) .vi"("AXI4-Stream Reader FXP64x4"=w275, "ready for output"=TRUE) -> ("data"=w276:bool[], "output valid"=w277:bool)  [unwired: 12 in]
    n158 = And(x=w277, y="aurora.read port 4") -> (x .and. y?=w279:bool)
    n159 = case shown="True" w279 {
      tunnel: w276 -> [_ w293]
      tunnel: [FALSE ("Timed Out?") w292] -> w274
      frame False {
      }
      frame True {
        n160 = disable-structure shown="Disabled" {
          disable-tunnel: w293 -> [w296 _]
          disable-tunnel: [w295 _] -> w292
          frame Disabled {
            n161 = xnode ("FIFO Method Node")("Element"=w296, "Timeout"=0) -> ("Timed Out?"=w295:bool)  [unwired: 1 in, 1 out]
          }
          frame Enabled {
          }
        }
      }
    }
    n162 = call <instrlib>:"Synchronous Latch.vi"("clear"="port 4.rx fifo overflow clear", "set"=w274) -> ("out"=→"port 4.rx fifo overflow":bool)  [unwired: 9 in]
    n163 = feedback #15(FALSE ("ready for input")) -> (w283:bool)
    n164 = case shown="True" w283 {
      tunnel: [_ w300] -> w289
      tunnel: [TRUE ("Timed Out?") w299] -> w286
      frame False {
      }
      frame True {
        n165 = xnode ("FIFO Method Node")("Timeout"=0) -> ("Element"=w300:bool[], "Timed Out?"=w299:bool)  [unwired: 1 in, 1 out]
      }
    }
    n166 = call "Aurora Read Debug Signals (Single Port).vi"("Debug CLIP Resources"=T27 {"Hard Error"="7902R IO Socket\\uPort4_HardError", "Soft Error"="7902R IO Socket\\uPort4_SoftError", "Lane Up"="7902R IO Socket\\uPort4_LaneUp", "Channel Up"="7902R IO Socket\\uPort4_ChannelUp", "Sys Reset"="7902R IO Socket\\uPort4_sys_reset_out"}) -> ("Debug Info"=→"port 4.debug info":T2)  [unwired: 14 in]
    n167 = Not(x=w286) -> (.not. x?=w285:bool)
    n168 = call "Aurora Writer (Single Port).vi"("input data"=w289, "AXI4-Stream Writer FXP64x4"=w290, "input valid"=w285) -> ("ready for input"=w284:bool)  [unwired: 12 in]
    n169 = feedback-in #15(w284) -> ()
  }
  n170 = node-c288(w32) -> ()
  n171 = node-c288(w7) -> ()
  n172 = node-c288(w5) -> ()
  n173 = node-c288(w30) -> ()
